vi "practiceImageAnalysis20vi.vi"() -> ()   [LabVIEW 2016]
uses:
  <vilib>/vision/Measure.llb/Straight Edge Options.ctl
  <vilib>/vision/Measure.llb/Straight Edge Process.ctl
  <vilib>/vision/Measure.llb/Edge Options.ctl
  <vilib>/vision/Measure.llb/Edge Polarity.ctl
  <vilib>/Math Plots/2D Math Plots/2D Error Bar/2D Error Bar XCtrl/2D Error Bar.xctl
  <vilib>/Math Plots/2D Math Plots/2D Error Bar/2D Error Bar Datatype/Public/Plot Helper (Fixed).vi
  <vilib>/Utility/file.llb/Write Delimited Spreadsheet (DBL).vi
  <vilib>/regexp/Match Regular Expression.xnode
  <vilib>/Math Plots/2D Math Plots/2D Error Bar/2D Error Bar Datatype/2D Error Bar Datatype.lvclass
panel:
  out "Top SD":dbl[][](array[numeric])
  out "Bottom SD":dbl[][](array[numeric])
  out "Bottom averages":dbl[][](array[numeric])
  out "Top averages":dbl[][](array[numeric])
  out "Coords of points Bar":refnum<class "2D Plot Datatype.lvclass">[](xcontrol)
  out "Coordinate array for image capture":dbl[][](array[numeric])
  in  "Coordinate file for image capture":path=path "E:/XYZstage+Camera_CollectedImages/12-16-2016/noStaveMount/toolingpinsCoordinates-captured.csv"
  out "Review":bool
  out "Search running?":bool
  in  "Options: Bottom Edge Search":T3={"Search Direction"=3, "Edge Options"={"Edge Polarity"=2, "Kernel Size"=9, "Width"=3, "Minimum Edge Strength"=17.0, "Interpolation Type"=enum."Bilinear Fixed", "Data Processing Method"=enum."Average"}, "Show Search Area"=TRUE, "Show Search Lines"=TRUE, "Show Edges Found"=TRUE, "Show Result"=TRUE, "Search Area Color"=65280, "Search Lines Color"=255, "Edge Locations Color"=16776960, "Result Color"=16711680, "Overlay Group Name"=""} {"Search Direction" items=["Left to Right", "Right to Left", "Top to Bottom", "Bottom to Top"]; "Edge Options"."Edge Polarity" items=["All Edges", "Rising Edges", "Falling Edges"]; "Edge Options"."Minimum Edge Strength" format="%.2f"; "Edge Options"."Width" step=2; "Edge Options"."Kernel Size" step=2}
  in  "Options: Top Edge Search":T3={"Search Direction"=2, "Edge Options"={"Edge Polarity"=0, "Kernel Size"=5, "Width"=3, "Minimum Edge Strength"=16.0, "Interpolation Type"=enum."Bilinear Fixed", "Data Processing Method"=enum."Average"}, "Show Search Area"=TRUE, "Show Search Lines"=TRUE, "Show Edges Found"=TRUE, "Show Result"=TRUE, "Search Area Color"=65280, "Search Lines Color"=255, "Edge Locations Color"=16776960, "Result Color"=16711680, "Overlay Group Name"=""} {"Search Direction" items=["Left to Right", "Right to Left", "Top to Bottom", "Bottom to Top"]; "Edge Options"."Edge Polarity" items=["All Edges", "Rising Edges", "Falling Edges"]; "Edge Options"."Minimum Edge Strength" format="%.2f"; "Edge Options"."Width" step=2; "Edge Options"."Kernel Size" step=2}
  in  "Fit Options":T4={"Number of Lines"=1, "Type"=enum."First Edge Rake", "Min. Score"=10.0, "Max. Score"=1000.0, "Orientation"=0.0, "Angle Range"=45.0, "Angle Tolerance"=1.0, "Step Size"=196, "Min. SNR (db)"=0.0, "Min. Points (%)"=25.0, "Hough Iterations"=5} {"Min. Points (%)" min=0.0 max=100.0; "Min. SNR (db)" min=0.0; "Max. Score" min=0.0 max=1024.0; "Min. Score" min=0.0 max=1024.0 step=1.0}
  in  "Stop and delete":bool
  out "Images Array":T6[](array[plugin-control])
  in  "error in":errorcluster
  out "error out":errorcluster
  out "Filenames Array":string[](array[string])
  in  "Naming Convention":string="*.png"
  in  "Images Directory":path=path "E:/XYZstage+Camera_CollectedImages/12-16-2016/noStaveMount/toolingpins_images"
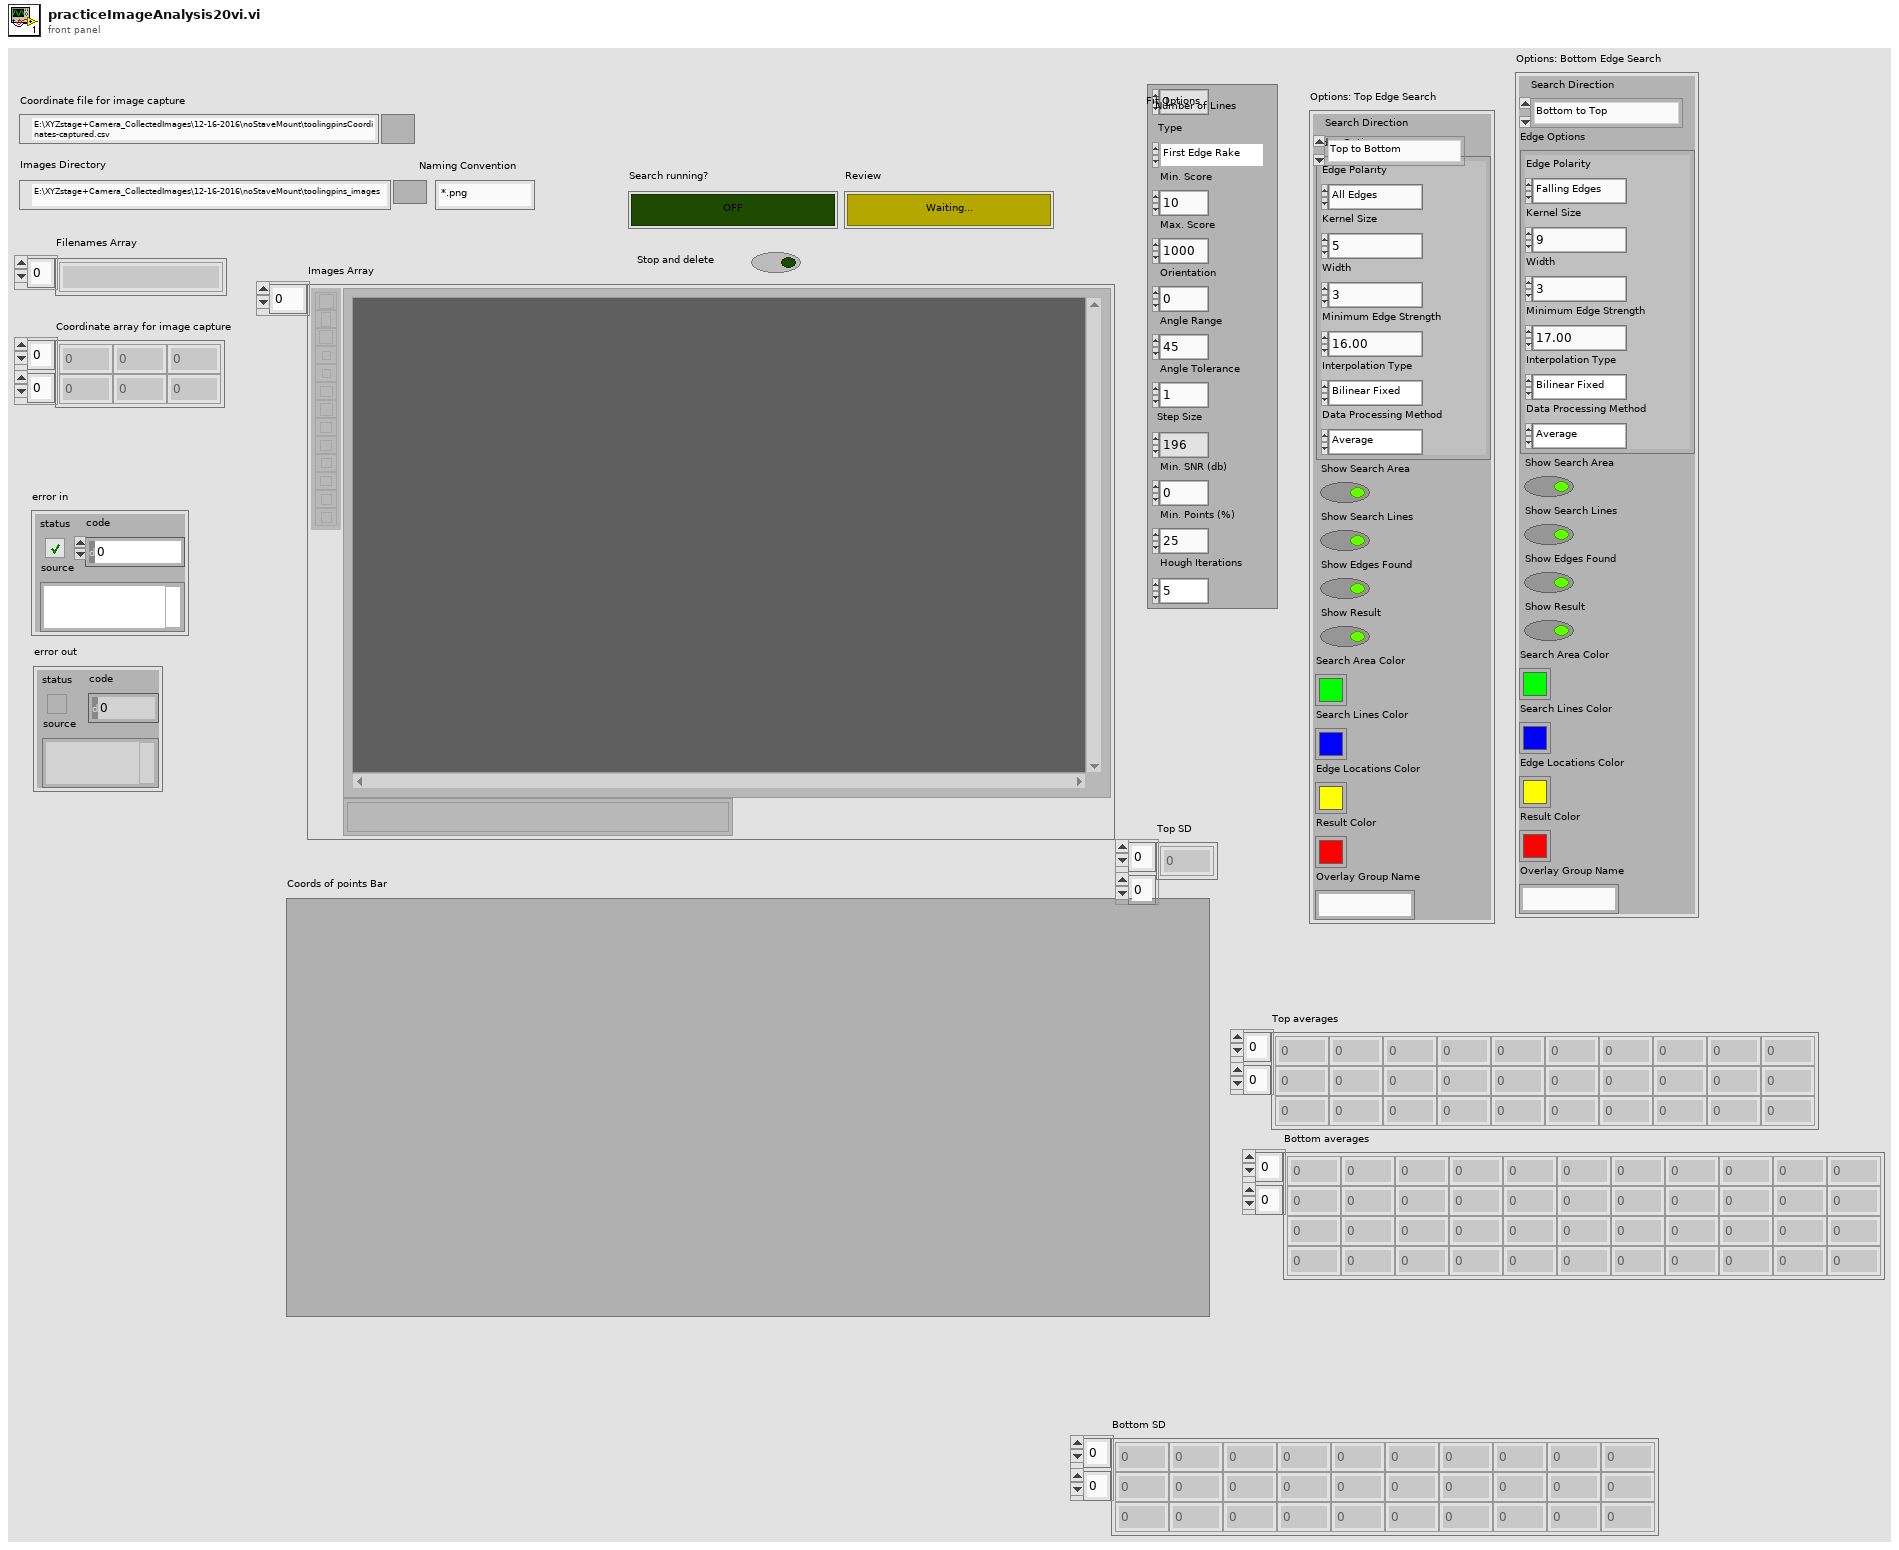
[diagram p1: front panel]
types:
  T1 = typedef "Edge Options.ctl" = cluster{"Edge Polarity":T2, "Kernel Size":u32, "Width":u32, "Minimum Edge Strength":sgl, "Interpolation Type":enum32{"Zero Order", "Bilinear", "Quadratic", "Cubic", "Bilinear Fixed"}, "Data Processing Method":enum32{"Average", "Median"}}
  T2 = typedef "Edge Polarity.ctl" = u32
  T3 = cluster{"Search Direction":u32, "Edge Options":T1, "Show Search Area":bool, "Show Search Lines":bool, "Show Edges Found":bool, "Show Result":bool, "Search Area Color":u32, "Search Lines Color":u32, "Edge Locations Color":u32, "Result Color":u32, "Overlay Group Name":string}
  T4 = typedef "Straight Edge Options.ctl" = cluster{"Number of Lines":i32, "Type":T5, "Min. Score":dbl, "Max. Score":dbl, "Orientation":dbl, "Angle Range":dbl, "Angle Tolerance":dbl, "Step Size":u32, "Min. SNR (db)":dbl, "Min. Points (%)":dbl, "Hough Iterations":i32}
  T5 = typedef "Straight Edge Process.ctl" = enum32{"First Edge Rake", "Best Edge Rake", "Hough Edge Rake", "First Edge Projection", "Best Edge Projection"}
  T6 = typedef "IMAQ Image.ctl" = refnum<image>
  T7 = enum16{"cm", "mm", "pixels [mm/pix]", "pixels [um/pix]"}
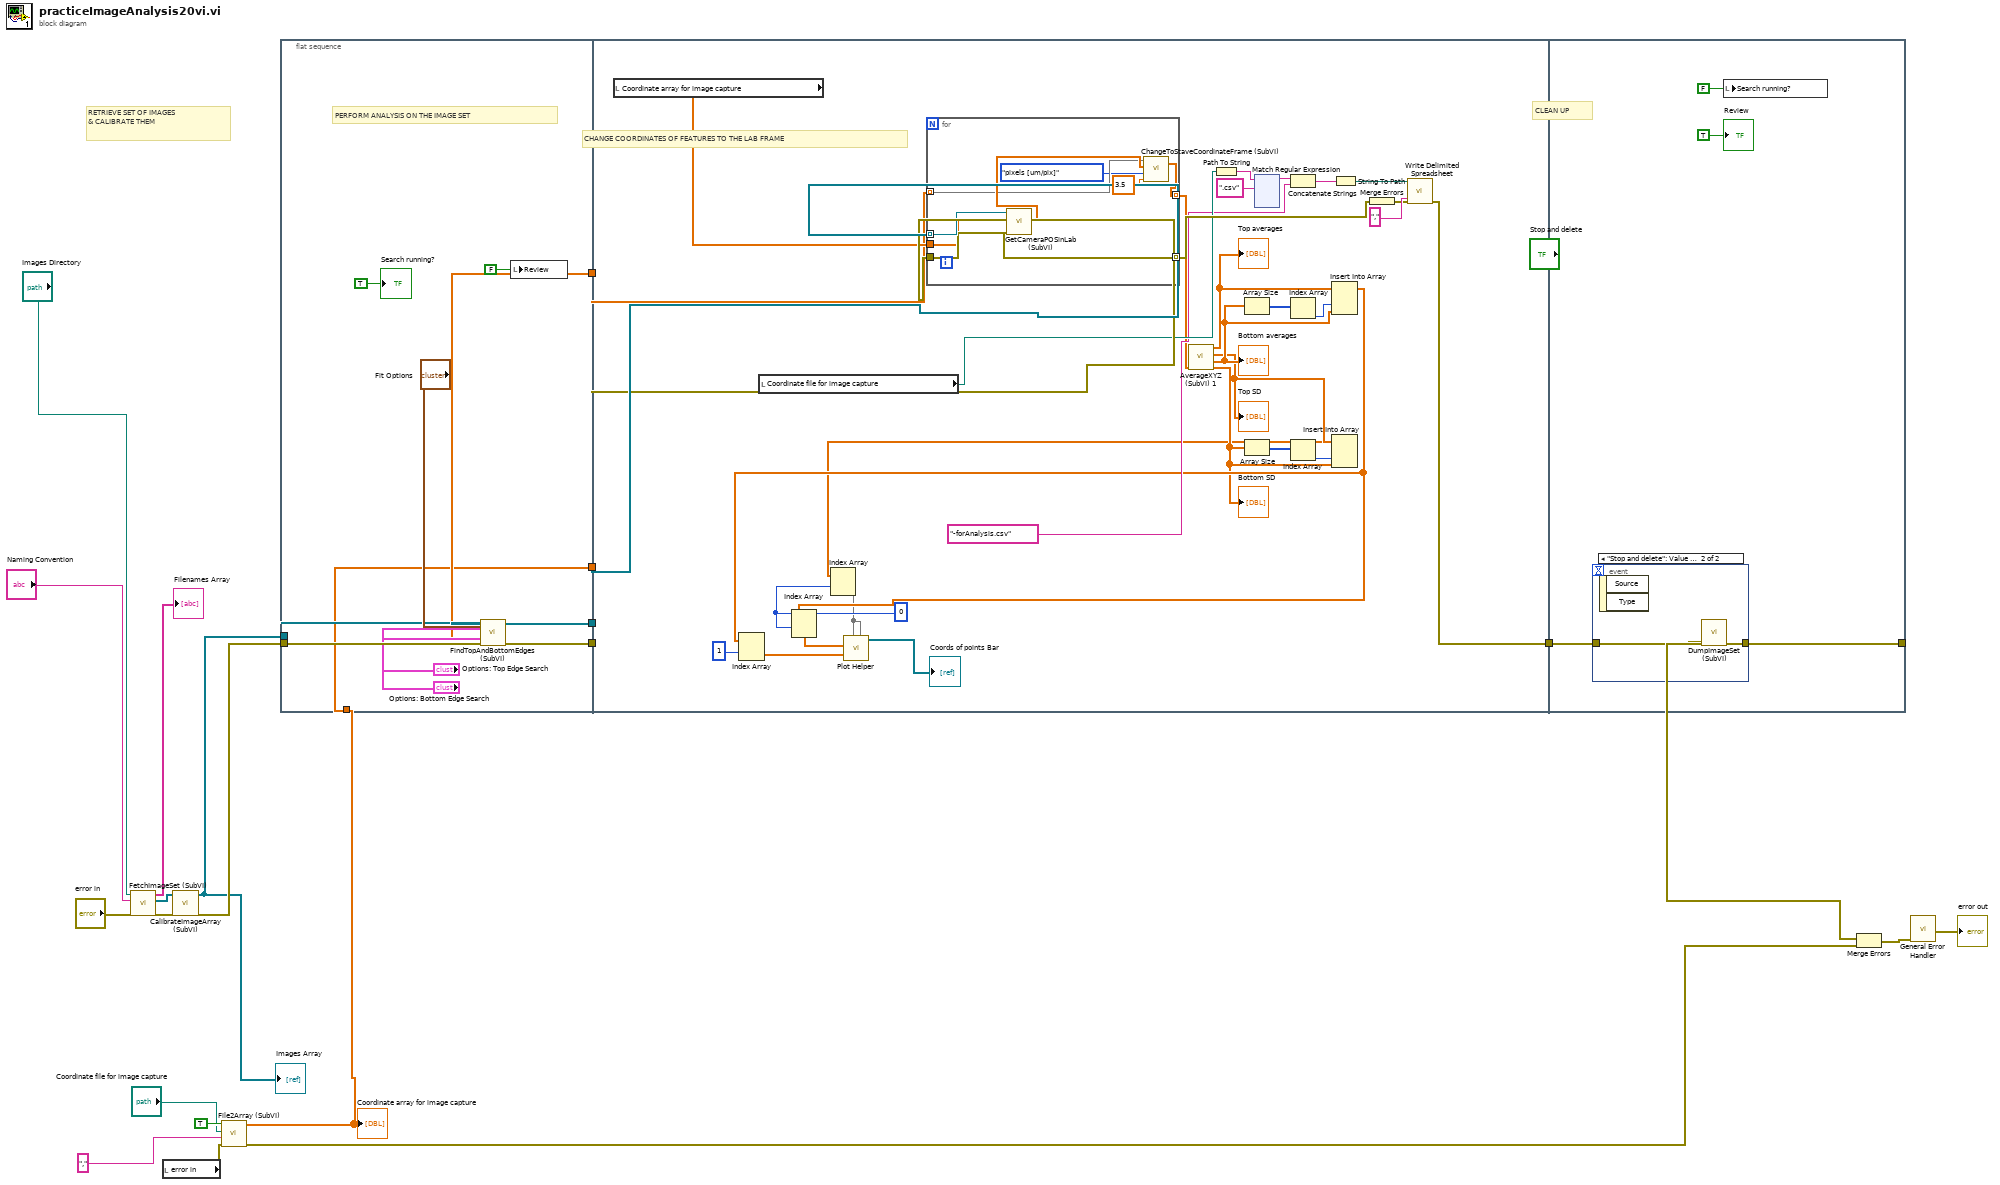
[diagram p0: block diagram]
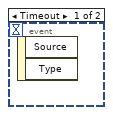
[diagram p2: hidden frame]
diagram:
  # "RETRIEVE SET OF IMAGES\n& CALIBRATE THEM"
  n1 = call "FetchImageSet (SubVI).vi"("error in (no error)"="error in", "Naming Convention"="Naming Convention", "Images Directory"="Images Directory") -> ("error out"=w18:errorcluster, "Image Array"=w19:T6[], "Filenames Array"=→"Filenames Array":string[])  [unwired: 6 in]
  n2 = local read "error in"() -> (w8:errorcluster)
  n3 = call "CalibrateImageArray (SubVI).vi"("error in (no error)"=w18, "Image Array"=w19) -> ("error out"=w15:errorcluster, "Calibrated Image Array"=w14:T6[])  [unwired: 7 in]
  "Images Array" <- w14
  n4 = call "File2Array (SubVI).vi"("error in (no error) in"=w8, "File delimiter"=",", "Source array file"="Coordinate file for image capture", "Load array from file?"=TRUE) -> ("error in (no error) out"=w6:errorcluster, "Loaded array"=w2:dbl[][])  [unwired: 6 in]
  "Coordinate array for image capture" <- w2
  n5 = flat-sequence {
    tunnel: w15 -> [w33]
    tunnel: w14 -> [w25]
    tunnel: [w32] -> w13
    tunnel: [w31] -> w12
    tunnel: [w24] -> w4
    tunnel: w2 -> [w23]
    tunnel: [w23] -> w1
    tunnel: w13 -> [w64]
    tunnel: w12 -> [w65]
    tunnel: w4 -> [w62]
    tunnel: [w51] -> w3
    tunnel: w1 -> [_]
    tunnel: [w190] -> w7
    tunnel: w3 -> [w189]
    frame #0 {
      # "PERFORM ANALYSIS ON THE IMAGE SET"
      n6 = call "FindTopAndBottomEdges (SubVI).vi"("Calibrated Image Array"=w25, "Fit Options"="Fit Options", "Options: Top Edge Search"="Options: Top Edge Search", "Options: Bottom Edge Search"="Options: Bottom Edge Search", "error in (no error)"=w33) -> ("Analyzed Image Array"=w31:T6[], "Array of Edge Endpoint Arrays"=w24:sgl[][][], "error out"=w32:errorcluster)  [unwired: 6 in, 2 out]
      n7 = local write "Review"(FALSE ("Review")) -> ()
      "Search running?" <- TRUE ("Search running?")
    }
    frame #1 {
      w47 = 0 ("index (row)")
      # "CHANGE COORDINATES OF FEATURES TO THE LAB FRAME"
      n8 = local read "Coordinate array for image capture"() -> (w63:dbl[][])
      n9 = local read "Coordinate file for image capture"() -> (w60:path)
      n10 = for {
        tunnel: w65 -> [w188] mode=indexing
        tunnel: w64 -> [w187]
        tunnel: w63 -> [w186]
        tunnel: w62 -> [w184] mode=indexing
        tunnel: [w181] -> w61 mode=indexing
        tunnel: [w180] -> w50 mode=indexing
        n11 = call "GetCameraPOSinLab (SubVI).vi"("error in (no error)"=w187, "Loaded array"=w186, "Refnum in"=w188) -> ("error out"=w181:errorcluster, "Image coordinates in lab frame"=w185:dbl[])  [unwired: 6 in, 1 out]
        n12 = call "ChangeToStaveCoordinateFrame (SubVI).vi"("Loaded array (image frame)"=w184, "Image Origin in XYZ Stage Coords [mm]"=w185, "Units"=T7."pixels [um/pix]", "Pixel resolution"=3.5) -> ("Array (stage frame, mm)"=w180:dbl[][])  [unwired: 2 in]
      }
      n13 = call "AverageXYZ (SubVI) 1.vi"("array"=w50) -> ("Bottom SD"=w36:dbl[][], "Bottom averages"=w45:dbl[][], "Top SD"=w39:dbl[][], "Top averages"=w46:dbl[][])  [unwired: 7 in]
      "Top averages" <- w46
      "Bottom averages" <- w45
      "Bottom SD" <- w36
      "Top SD" <- w39
      n14 = Path To String(path=w60) -> (string=w58:string)
      n15 = Array Size(array=w45) -> (size(s)=w44:i32[])
      n16 = Array Size(array=w36) -> (size(s)=w37:i32[])
      n17 = xnode "Match Regular Expression"("input string"=w58, "regular expression"=".csv") -> ("before match"=w56:string)  [unwired: 4 in, 4 out]
      n18 = Concatenate Strings(w56, "-forAnalysis.csv" ("name or relative path")) -> (w55:string)
      n19 = Index Array(array=w44) -> (element=w43:i32)  [unwired: 1 in]
      n20 = Index Array(array=w37) -> (element=w38:i32)  [unwired: 1 in]
      n21 = Insert Into Array(array=w46, index (col)=w43, new element=w45) -> (w42:dbl[][])  [unwired: 1 in]
      n22 = Index Array(array=w42, index (row)=1) -> (element=w40:dbl[])  [unwired: 1 in]
      n23 = Index Array(array=w42, index (row)=w47) -> (element=w41:dbl[])  [unwired: 1 in]
      n24 = Insert Into Array(array=w39, index (col)=w38, new element=w36) -> (w35:dbl[][])  [unwired: 1 in]
      n25 = Index Array(array=w35, index (row)=w47) -> (element=w34:dbl[])  [unwired: 1 in]
      n26 = call-poly <vilib>:"Plot Helper.vi"("error b vector"=w34, "error a vector"=w34, "y vector"=w40, "x vector"=w41) -> ("2D Plot Class Obj Array out"=→"Coords of points Bar":refnum<class "2D Plot Datatype.lvclass">[])  [unwired: 2 in, 5 out]
      n27 = String To Path(string=w55) -> (path=w53:path)
      n28 = Merge Errors(w61) -> (w52:errorcluster)
      n29 = call-poly <vilib>:"Write Delimited Spreadsheet.vi"("file path (dialog if empty)"=w53, "error in (no error)"=w52, "delimiter (\\t)"="," ("delimiter (\\t)")) -> ("error out"=w51:errorcluster)  [unwired: 11 in, 1 out]
    }
    frame #2 {
      # "CLEAN UP"
      n30 = event shown="[1] \"Stop and delete\": Value Change" {
        selector: _ -> [_ _]
        dyn-events: _ -> [_ _]
        timeout: _ -> [_ _]
        tunnel: [_ w194] -> w190
        tunnel: w189 -> [_ w193]
        event Timeout {
          n31 = event-data() -> ()  [unwired: 1 in, 2 out]
        }
        event "Stop and delete": Value Change {
          n32 = event-data() -> ()  [unwired: 1 in, 2 out]
          n33 = call "DumpImageSet (SubVI).vi"("error in (no error)"=w193) -> ("error out"=w194:errorcluster)  [unwired: 7 in]
        }
      }
      n34 = local write "Search running?"(FALSE ("Search running?")) -> ()
      "Review" <- TRUE ("Review")
    }
  }
  n35 = Merge Errors(w7, w6) -> (w5:errorcluster)
  n36 = call <vilib>:"General Error Handler.vi"("error in (no error)"=w5) -> ("error out"=→"error out":errorcluster)  [unwired: 10 in, 4 out]
